vi "FlatToRichexternal_driver_wrapper_CloseRequest.vi"(5 "OutputClusterType":T1, 11 "InputCluster":T2) -> (3 "OutputCluster":T1)   [LabVIEW 2020, in "Instrument Interaction Client.lvlib"]
uses:
  external_driver_wrapper_CloseRequest_Flat.ctl
  external_driver_wrapper_CloseRequest.ctl
  Instrument Interaction Client.lvlib
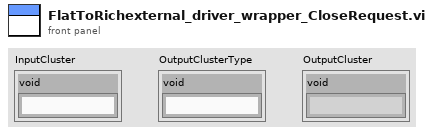
[diagram p1: front panel]
types:
  T1 = typedef "Instrument Interaction Client.lvlib/external_driver_wrapper_CloseRequest.ctl" = cluster{"void":string}
  T2 = typedef "Instrument Interaction Client.lvlib/external_driver_wrapper_CloseRequest_Flat.ctl" = cluster{"void":string}
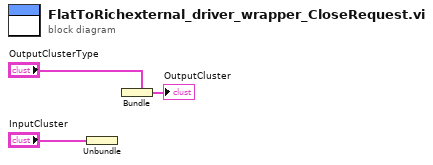
[diagram p0: block diagram]
diagram:
  n1 = Unbundle "Unbundle"("InputCluster") -> ()  [unwired: 1 out]
  n2 = Bundle "Bundle"(cluster="OutputClusterType") -> (→"OutputCluster":T1)  [unwired: 1 in]
